vi "myDAQ Action Engine.vi"(8 "Error In":errorcluster, 10 "Controller Output":T1, 11 "Enum Defining myDAQ Action":T3) -> (0 "Error Out":errorcluster, 2 "Inputs":T2)   [LabVIEW 2018]
doc: "This VI controls the operation of the myDAQ digital input and output llnes."
uses:
  controls/Enum Defining myDAQ Actions.ctl
  controls/Cluster for displaying  ABR switch states.ctl
  controls/Cluster for displaying  LED outputs.ctl
  <vilib>/DAQmx/read.llb/DAQmx Read (Digital 1D Bool 1Chan 1Samp).vi
  <vilib>/DAQmx/write.llb/DAQmx Write (Digital 1D Bool 1Chan 1Samp).vi
  <vilib>/DAQmx/create/channels.llb/DAQmx Create Channel (DO-Digital Output).vi
  <vilib>/DAQmx/create/channels.llb/DAQmx Create Channel (DI-Digital Input).vi
  <vilib>/DAQmx/miscellaneous.llb/DAQmx Fill In Error Info.vi
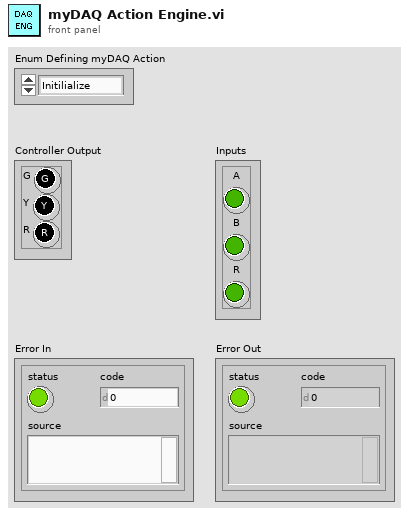
[diagram p1: front panel]
types:
  T1 = typedef "Cluster for displaying  LED outputs.ctl" = cluster{"G":bool, "Y":bool, "R":bool}
  T2 = typedef "Cluster for displaying  ABR switch states.ctl" = cluster{"A":bool, "B":bool, "R":bool}
  T3 = typedef "Enum Defining myDAQ Actions.ctl" = enum16{"Initilialize", "Read Buttons", "Set LED Lights", "Release"}
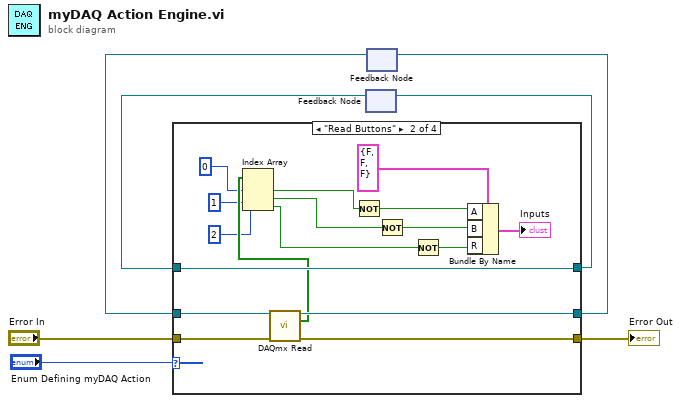
[diagram p0: block diagram]
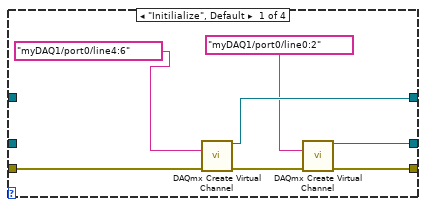
[diagram p2: hidden frame]
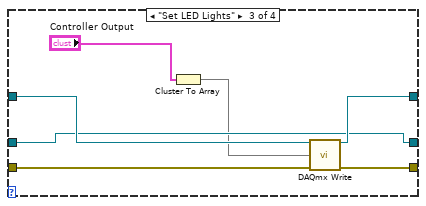
[diagram p3: hidden frame]
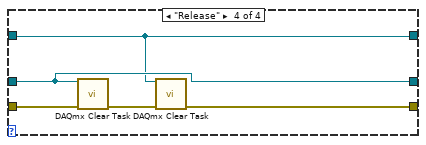
[diagram p4: hidden frame]
diagram:
  n1 = feedback #1() -> (w3:refnum<k21>)  [unwired: 1 in]
  n2 = feedback #2() -> (w1:refnum<k21>)  [unwired: 1 in]
  n3 = case shown="\"Read Buttons\"" "Enum Defining myDAQ Action" {
    tunnel: [w13 w29 w34 w40] -> w2
    tunnel: "Error In" -> [w12 w31 w38 w43]
    tunnel: [w11 w30 w37 w41] -> w5
    tunnel: [w10 w28 w35 w39] -> w4
    tunnel: w3 -> [_ w28 w36 w39]
    tunnel: w1 -> [_ w25 w34 w40]
    frame "Initilialize", Default {
      n4 = call-poly <vilib>:"DAQmx Create Virtual Channel.vi"("lines"=tag "myDAQ1/port0/line4:6", "error in"=w12) -> ("task out"=w10:refnum<k21>, "error out"=w14:errorcluster)  [unwired: 12 in]
      n5 = call-poly <vilib>:"DAQmx Create Virtual Channel.vi"("lines"=tag "myDAQ1/port0/line0:2", "error in"=w14) -> ("task out"=w13:refnum<k21>, "error out"=w11:errorcluster)  [unwired: 12 in]
    }
    frame "Read Buttons" {
      n6 = call-poly <vilib>:"DAQmx Read.vi"("task/channels in"=w25, "error in"=w31) -> ("task out"=w29:refnum<k21>, "data"=w24:bool[], "error out"=w30:errorcluster)  [unwired: 11 in]
      n7 = Index Array(array=w24, index #1=0 ("index"), index #2=1 ("index"), index #3=2 ("index")) -> (element #1=w15:bool, element #2=w16:bool, element #3=w17:bool)
      n8 = Not(x=w15) -> (.not. x?=w20:bool)
      n9 = Not(x=w16) -> (.not. x?=w19:bool)
      n10 = Not(x=w17) -> (.not. x?=w18:bool)
      n11 = Bundle By Name(cluster=T2 {"A"=FALSE, "B"=FALSE, "R"=FALSE} ("Inputs"), "A"=w20, "B"=w19, "R"=w18) -> (→"Inputs":T2)
    }
    frame "Set LED Lights" {
      n12 = Cluster To Array(cluster="Controller Output") -> (array=w33:bool[])
      n13 = call-poly <vilib>:"DAQmx Write.vi"("task/channels in"=w36, "data"=w33, "error in"=w38) -> ("task out"=w35:refnum<k21>, "error out"=w37:errorcluster)  [unwired: 10 in, 1 out]
    }
    frame "Release" {
      n14 = call <vilib>:"DAQmx Clear Task.vi"("task in"=w40, "error in"=w43) -> ("error out"=w42:errorcluster)  [unwired: 13 in]
      n15 = call <vilib>:"DAQmx Clear Task.vi"("task in"=w39, "error in"=w42) -> ("error out"=w41:errorcluster)  [unwired: 13 in]
    }
  }
  "Error Out" <- w5
  n16 = feedback-in #1(w4) -> ()
  n17 = feedback-in #2(w2) -> ()
